vi "ConfigTriggers.vi"(8 "error in (no error)":errorcluster, 11 "FgenPluginsBase in":refnum<class "FgenPluginsBase.lvclass">) -> (0 "error out":errorcluster, 3 "FgenPluginsBase out":refnum<class "FgenPluginsBase.lvclass">)   [LabVIEW 2014, in "FgenPlugins.lvlib" / "FgenPluginsBase.lvclass"]
uses:
  FgenPluginsBase.lvclass
  <userlib>/NIST/BaseClasses/Object_class/BaseObject.lvclass
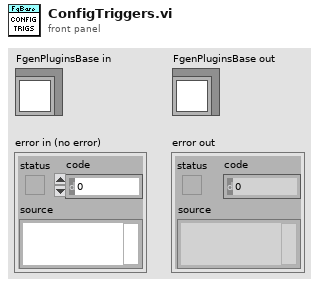
[diagram p1: front panel]
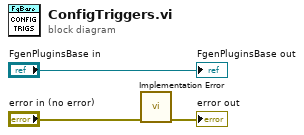
[diagram p0: block diagram]
diagram:
  n1 = call <userlib>:"Implementation Error.vi"("error in (no error)"="error in (no error)") -> ("error out"=→"error out":errorcluster)  [unwired: 10 in]
  "FgenPluginsBase out" <- "FgenPluginsBase in"
